vi "Save Global.vi"() -> ()   [LabVIEW 2017]
doc: "<b>Changes</b> the defaults of all controls on the front panel to be the current values. <b>Saves the VI</b>."
panel:
  in  "message":string="Save Global must be launched from the Global Variable VI you wish to save."
  # "Wait while we process you Global Variable VI.\n\nChanges the defaults of all controls on the front panel to be the current values. Saves the VI."
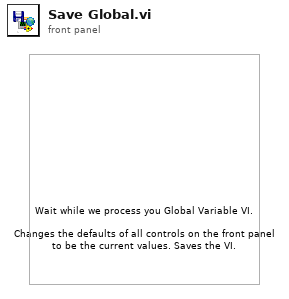
[diagram p1: front panel]
types:
  T1 = enum32{"Invalid", "Standard", "Closed", "Hidden", "Minimized", "Maximized"}
  T2 = enum32{"invalid VI type", "Standard VI", "Control VI", "Global VI", "Polymorphic VI", "Configuration VI", "SubSystem", "Facade VI", "Method VI", "Statechart Diagram VI"}
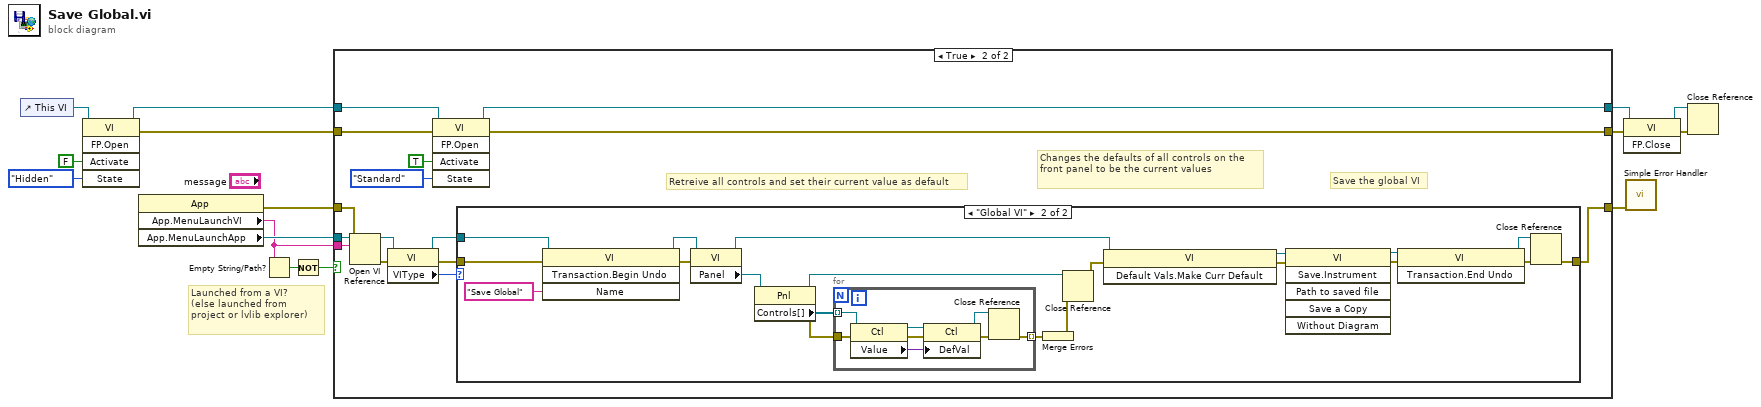
[diagram p0: block diagram]
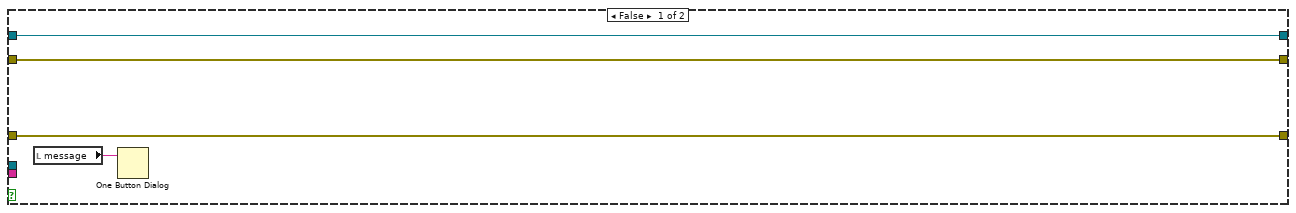
[diagram p2: hidden frame]
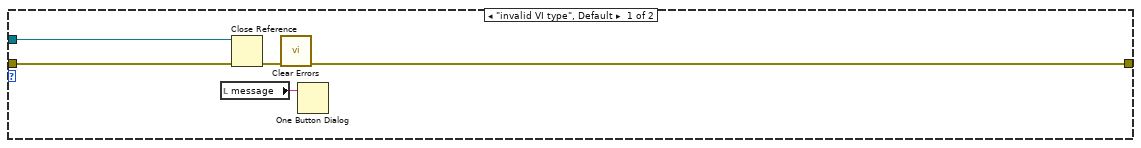
[diagram p3: hidden frame]
diagram:
  # "Launched from a VI?\n(else launched from project or lvlib explorer)"
  n1 = control-ref of="This VI"() -> (w1:refnum<vi>)
  n2 = invoke class="VI" method="FP.Open"(reference=w1, "Activate"=FALSE ("Activate?"), "State"=T1."Hidden") -> (reference out=w7:refnum<vi>, error out=w6:errorcluster)  [unwired: 2 in, 3 out]
  n3 = property class="App"() -> (error out=w14:errorcluster, "App.MenuLaunchVI"=w13:string, "App.MenuLaunchApp"=w15:refnum<vi>)  [unwired: 2 in, 1 out]
  n4 = Empty String/Path?(string/path=w13) -> (empty?=w12:bool)
  n5 = Not(x=w12) -> (.not. x?=w11:bool)
  n6 = case shown="True" w11 {
    tunnel: w15 -> [_ w34]
    tunnel: w14 -> [w19 w33]
    tunnel: w13 -> [_ w32]
    tunnel: [w19 w31] -> w10
    tunnel: w6 -> [w17 w24]
    tunnel: w7 -> [w16 w25]
    tunnel: [w17 w23] -> w8
    tunnel: [w16 w22] -> w9
    frame False {
      n7 = local read "message"() -> (w18:string)
      n8 = One Button Dialog(message=w18) -> ()  [unwired: 1 in, 1 out]
    }
    frame True {
      # "Save the global VI"
      # "Changes the defaults of all controls on the front panel to be the current values"
      # "Retreive all controls and set their current value as default"
      n9 = Open VI Reference(application reference (local)=w34, vi path=w32, error in (no error)=w33) -> (vi reference=w28:refnum<vi>, error out=w30:errorcluster)  [unwired: 3 in]
      n10 = property class="VI"(reference=w28, error in=w30) -> (reference out=w27:refnum<vi>, error out=w29:errorcluster, "VIType"=w26:T2)
      n11 = invoke class="VI" method="FP.Open"(reference=w25, error in=w24, "Activate"=TRUE ("Activate?"), "State"=T1."Standard") -> (reference out=w22:refnum<vi>, error out=w23:errorcluster)  [unwired: 1 in, 3 out]
      n12 = case shown="\"Global VI\"" w26 {
        tunnel: [w36 w59] -> w31
        tunnel: w29 -> [w39 w48]
        tunnel: w27 -> [w38 w45]
        frame "invalid VI type", Default {
          n13 = local read "message"() -> (w35:string)
          n14 = Close Reference(reference=w38, error in (no error)=w39) -> (error out=w37:errorcluster)
          n15 = call <vilib>:"Clear Errors.vi"("error in (no error)"=w37) -> ("error out"=w36:errorcluster)  [unwired: 5 in, 1 out]
          n16 = One Button Dialog(message=w35) -> ()  [unwired: 1 in, 1 out]
        }
        frame "Global VI" {
          n17 = invoke class="VI" method="Transaction.Begin Undo"(reference=w45, error in=w48, "Name"="Save Global") -> (reference out=w46:refnum<vi>, error out=w47:errorcluster)  [unwired: 1 in, 2 out]
          n18 = property class="VI"(reference=w46, error in=w47) -> (reference out=w51:refnum<vi>, "Panel"=w58:refnum<vi>)  [unwired: 1 out]
          n19 = property class="Pnl"(reference=w58) -> (reference out=w55:refnum<vi>, error out=w56:errorcluster, "Controls[]"=w57:refnum<vi>[])  [unwired: 1 in]
          n20 = for {
            tunnel: w57 -> [w61] mode=indexing
            tunnel: [w64] -> w54 mode=indexing
            tunnel: w56 -> [w60]
            n21 = property class="Ctl"(reference=w61, error in=w60) -> (reference out=w67:refnum<vi>, error out=w65:errorcluster, "Value"=w66:variant)
            n22 = property class="Ctl"(reference=w67, error in=w65, "DefVal"=w66) -> (reference out=w62:refnum<vi>, error out=w63:errorcluster)
            n23 = Close Reference(reference=w62, error in (no error)=w63) -> (error out=w64:errorcluster)
          }
          n24 = Merge Errors(w54) -> (w53:errorcluster)
          n25 = Close Reference(reference=w55, error in (no error)=w53) -> (error out=w52:errorcluster)
          n26 = invoke class="VI" method="Default Vals.Make Curr Default"(reference=w51, error in=w52) -> (reference out=w50:refnum<vi>, error out=w49:errorcluster)  [unwired: 1 in, 1 out]
          n27 = invoke class="VI" method="Save.Instrument"(reference=w50, error in=w49) -> (reference out=w43:refnum<vi>, error out=w42:errorcluster)  [unwired: 4 in, 4 out]
          n28 = invoke class="VI" method="Transaction.End Undo"(reference=w43, error in=w42) -> (reference out=w40:refnum<vi>, error out=w41:errorcluster)  [unwired: 1 in, 1 out]
          n29 = Close Reference(reference=w40, error in (no error)=w41) -> (error out=w59:errorcluster)
        }
      }
    }
  }
  n30 = invoke class="VI" method="FP.Close"(reference=w9, error in=w8) -> (reference out=w2:refnum<vi>, error out=w3:errorcluster)  [unwired: 1 in, 1 out]
  n31 = call <vilib>:"Simple Error Handler.vi"("error in (no error)"=w10) -> ()  [unwired: 4 in, 5 out]
  n32 = Close Reference(reference=w2, error in (no error)=w3) -> ()  [unwired: 1 out]
